vi "Config Write Sidestep Globals.vi"(11 "refnum":T1) -> (3 "refnum 2":T1)   [LabVIEW 2012]
uses:
  <vilib>/Utility/config.llb/Config Data RefNum.ctl
  Sidestep Globals.vi
  <vilib>/Utility/config.llb/Write Key (Double).vi
  <vilib>/Utility/config.llb/NI_LVConfig.lvlib
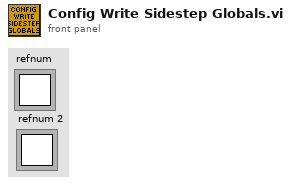
[diagram p1: front panel]
types:
  T1 = typedef "NI_LVConfig.lvlib/Config Data RefNum.ctl" = refnum<k1>
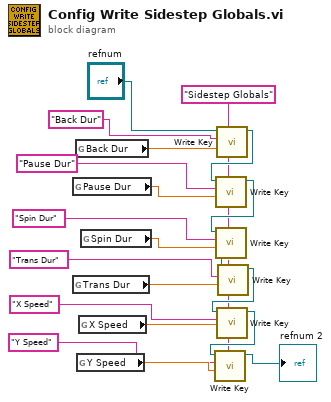
[diagram p0: block diagram]
diagram:
  w2 = "Sidestep Globals"
  n1 = global read "Sidestep Globals.vi" "Pause Dur"() -> (w16:dbl)
  n2 = global read "Sidestep Globals.vi" "Trans Dur"() -> (w12:dbl)
  n3 = global read "Sidestep Globals.vi" "Back Dur"() -> (w20:dbl)
  n4 = global read "Sidestep Globals.vi" "Y Speed"() -> (w10:dbl)
  n5 = global read "Sidestep Globals.vi" "X Speed"() -> (w11:dbl)
  n6 = global read "Sidestep Globals.vi" "Spin Dur"() -> (w15:dbl)
  n7 = call-poly <vilib>:"Write Key.vi"("section"=w2, "value"=w20, "key"="Back Dur", "refnum"="refnum") -> ("refnum out"=w18:T1)  [unwired: 5 in, 2 out]
  n8 = call-poly <vilib>:"Write Key.vi"("section"=w2, "value"=w16, "key"="Pause Dur", "refnum"=w18) -> ("refnum out"=w17:T1)  [unwired: 5 in, 2 out]
  n9 = call-poly <vilib>:"Write Key.vi"("section"=w2, "value"=w15, "key"="Spin Dur", "refnum"=w17) -> ("refnum out"=w14:T1)  [unwired: 5 in, 2 out]
  n10 = call-poly <vilib>:"Write Key.vi"("section"=w2, "value"=w12, "key"="Trans Dur", "refnum"=w14) -> ("refnum out"=w13:T1)  [unwired: 5 in, 2 out]
  n11 = call-poly <vilib>:"Write Key.vi"("section"=w2, "value"=w11, "key"="X Speed", "refnum"=w13) -> ("refnum out"=w9:T1)  [unwired: 5 in, 2 out]
  n12 = call-poly <vilib>:"Write Key.vi"("section"=w2, "value"=w10, "key"="Y Speed", "refnum"=w9) -> ("refnum out"=→"refnum 2":T1)  [unwired: 5 in, 2 out]
